vi "testsonar.vi"() -> ()   [LabVIEW 2019]
panel:
  in  "stop 2":bool
  in  "選擇超音波 2":enum16{"請選擇超音波", "超音波1", "超音波2", "超音波3", "超音波4"}(ring)
  out "公分 2":dbl
  out "公分":dbl
  in  "選擇超音波":enum16{"請選擇超音波", "超音波1", "超音波2", "超音波3", "超音波4"}(ring)
  in  "stop":bool
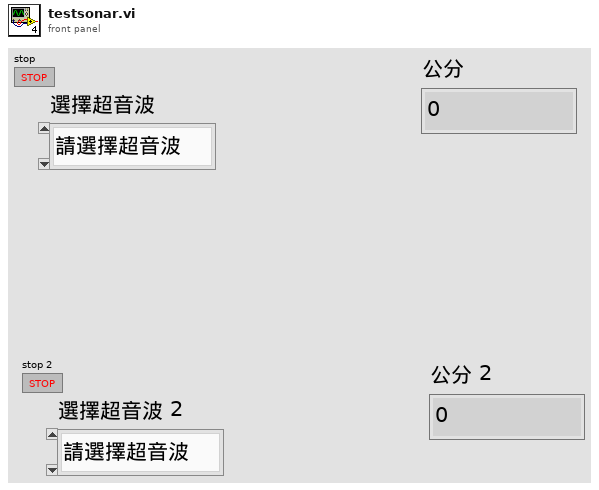
[diagram p1: front panel]
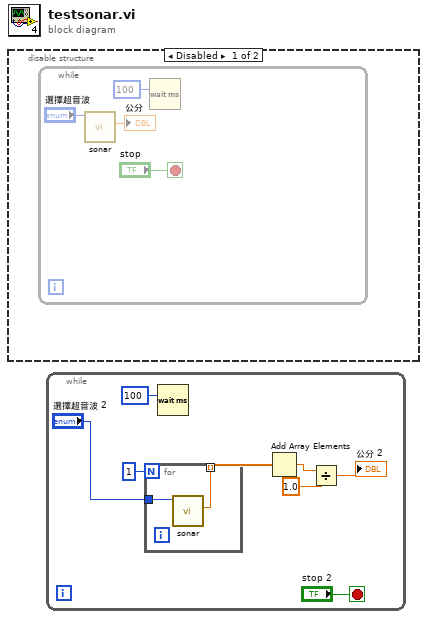
[diagram p0: block diagram]
diagram:
  n1 = disable-structure shown="Disabled" {
    frame Disabled {
      n2 = while {
        stop <- "stop" stop-if-true
        n3 = call "sonar.vi"("選擇超音波"="選擇超音波") -> ("公分"=→"公分":dbl)  [unwired: 9 in, 1 out]
        n4 = Wait (ms)(milliseconds to wait=u32 100) -> ()  [unwired: 1 out]
      }
    }
    frame Enabled {
    }
  }
  n5 = while {
    stop <- "stop 2" stop-if-true
    n6 = for {
      N: 1 -> [_]
      tunnel: "選擇超音波 2" -> [w14]
      tunnel: [w13] -> w8 mode=indexing
      n7 = call "sonar.vi"("選擇超音波"=w14) -> ("公分"=w13:dbl)  [unwired: 9 in, 1 out]
    }
    n8 = Wait (ms)(milliseconds to wait=u32 100) -> ()  [unwired: 1 out]
    n9 = Add Array Elements(numeric array=w8) -> (sum=w7:dbl)
    n10 = Divide(x=w7, y=1.0) -> (x/y=→"公分 2":dbl)
  }
